vi "AOL Z Range Calculation.vi"(9 "Current Objective":string, 10 "FOV values cluster":T1, 11 "FOV selection index":i32) -> (1 "AOL Z Range":dbl[](array[numeric]))   [LabVIEW 2020]
uses:
  Typedefs/FOV values cluster.ctl
  <vilib>/Utility/miscctls.llb/LVStringsAndValuesArrayTypeDef_SGL.ctl
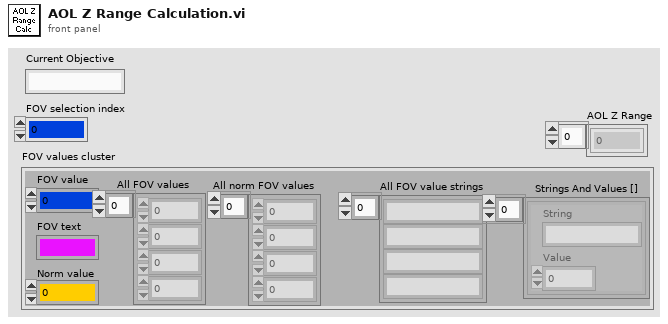
[diagram p1: front panel]
types:
  T1 = typedef "FOV values cluster.ctl" = cluster{"Norm value":sgl, "FOV text":string, "FOV value":i32, "All FOV values":i32[], "All norm FOV values":sgl[], "All FOV value strings":string[], "Strings And Values []":T2}
  T2 = typedef "LVStringsAndValuesArrayTypeDef_SGL.ctl" = cluster{"String":string, "Value":sgl}[]
  T3 = typedef "AOL_Globals.ctl" = cluster{"Imaging Protocol":T4, "Number of POI":u16, "Number of Miniscans":u16, "Number of Trials":u16, "Number of Cycles ":u64, "# Averaged Frames":u16, "Laser power (%)":u8, "Pockels (V)":dbl, "Acquisition Length (sec)":dbl, "Fill time (us)":dbl, "POI Dwell time (us)":dbl, "Miniscan Dwell time per pixel (us)":dbl, "PMT 1":dbl, "PMT 2":dbl, "Back Apperture (mA)":dbl, "Frame Size":T5, "Center Frequency":dbl, "Field of View (norm)":dbl, "DwellTime (us)":dbl, "Wavelength (nm)":dbl, "Zoom":dbl, "AOL Z":dbl, "AOL Mode":T6, "GridXY":dbl, "GridZ":dbl, "TriggerPeriod (sec)":dbl, "Number of Pixels in Miniscan":u16, "Experiment folder path":path, "X centre":dbl, "Y centre":dbl, "Angle (degrees)":dbl, "Plane Mode":T7, "Threshold":u16[], "Regenerate Chirps":bool, "Rectangle ROI length (pixels)":u16, "Rectangle ROI height (pixels)":u16, "AOD fill":u16, "StartupDelay":i32, "Samples Wait after Trigger":u16, "Slip Cycle":u32, "Add Cycle":bool, "Functional Mode":T8, "Z Start":dbl, "Z Stop":dbl, "# Planes":i32, "Total Pixels":i32, "Variable Miniscan Pixels":u16[], "Use Variable Length":bool, "Use Variable Resolution":bool, "Laser power (%) at Z Start":u8, "Laser power (%) at Z Stop":u8, "Ref Z Step":i8, "Ref Dwell Time (us)":dbl, "Field of View (um)":dbl}
  T4 = typedef "Imaging Protocols enum.ctl" = enum16{"AOL Z-Stack", "Motor Z Stack", "Functional Acquisition", "Single Plane Acquisition", "Volume Acquisition", "Live Imaging", "Live Plane Imaging", "Live Volume Imaging"}
  T5 = typedef "Frame Size.ctl" = u16
  T6 = typedef "AOL modes.ctl" = enum16{"Raster", "Structural", "Pointing", "Mini Scan", "Alignment"}
  T7 = typedef "Plane Mode.ctl" = u16
  T8 = typedef "Functional Mode.ctl" = enum16{"Point", "Line", "Patch", "Plane", "Volume"}
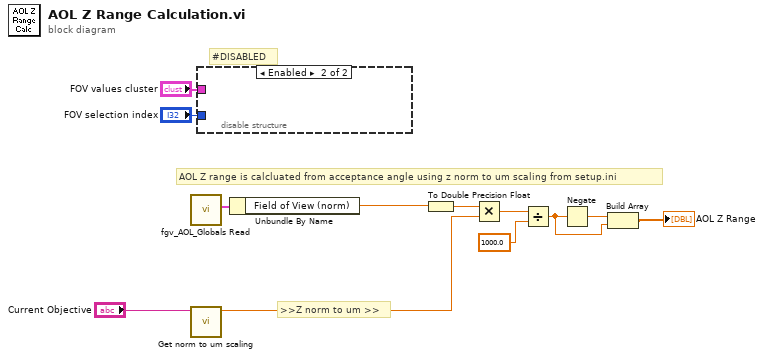
[diagram p0: block diagram]
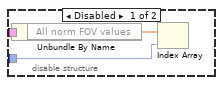
[diagram p2: hidden frame]
diagram:
  # "#DISABLED"
  # ">>Z norm to um >>"
  # "AOL Z range is calcluated from acceptance angle using z norm to um scaling from setup.ini"
  n1 = call "fgv_AOL_Globals Read.vi"() -> ("AOL_Globals"=w2:T3)  [unwired: 9 in, 2 out]
  n2 = call "Get norm to um scaling .vi"("Current Objective"="Current Objective") -> ("Z_norm to um_scaling"=w4:dbl)  [unwired: 7 in, 3 out]
  n3 = disable-structure shown="Enabled" {
    disable-tunnel: "FOV values cluster" -> [w15 _]
    disable-tunnel: "FOV selection index" -> [w13 _]
    frame Disabled {
      n4 = Unbundle By Name(w15) -> ("All norm FOV values"=w14:sgl[])
      n5 = Index Array(array=w14, index=w13) -> ()  [unwired: 1 out]
    }
    frame Enabled {
    }
  }
  n6 = Unbundle By Name(w2) -> ("Field of View (norm)"=w1:dbl)
  n7 = To Double Precision Float(number=w1) -> (double precision float=w10:dbl)
  n8 = Multiply(x=w10, y=w4) -> (x*y=w9:dbl)
  n9 = Divide(x=w9, y=1000.0) -> (x/y=w6:dbl)
  n10 = Negate(x=w6) -> (-x=w7:dbl)
  n11 = Build Array(w7, w6) -> (→"AOL Z Range":dbl[])
